vi "Replace tokens with underscore.vi"(11 "Sting":string) -> (3 "sanitized":string)   [LabVIEW 2019, in "SimpleDependencyInspector.lvlib"]
uses:
  SimpleDependencyInspector.lvlib
  <vilib>/Utility/error.llb/whitespace.ctl
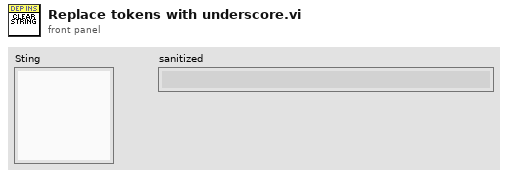
[diagram p1: front panel]
types:
  T1 = typedef "whitespace.ctl" = u16
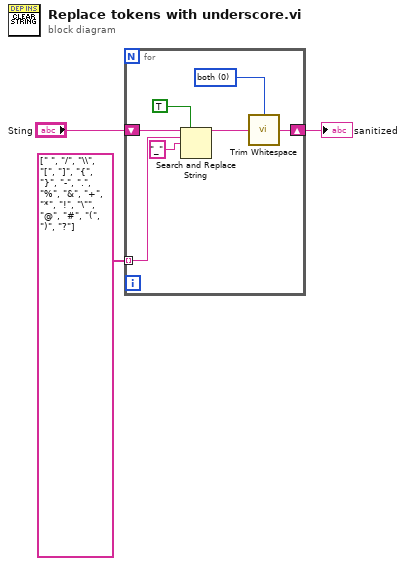
[diagram p0: block diagram]
diagram:
  n1 = for {
    shift-right: [w5] -> w2
    shift-left: "Sting" -> [w10]
    tunnel: string[] [" ", "/", "\\", "[", "]", "{", "}", "-", ".", "%", "&", "+", "*", "!", "\"", "@", "#", "(", ")", "?"] -> [w7] mode=indexing
    w4 = T1 0 items=["both", "start of string", "end of string"] ("location (both)")
    n2 = Search and Replace String(replace all?=TRUE ("replace all? (F)"), input string=w10, search string=w7, replace string="_" ("replace string (\"\")")) -> (result string=w6:string)  [unwired: 4 in, 3 out]
    n3 = call <vilib>:"Trim Whitespace.vi"("string"=w6, "location (both)"=w4) -> ("trimmed string"=w5:string)
  }
  "sanitized" <- w2
